vi "统计信息.vi"() -> ()   [LabVIEW 2016]
uses:
  <vilib>/Analysis/baseanly.llb/Mean (DBL).vi
  <vilib>/Analysis/NI_AALBase.lvlib
panel:
  in  "退出":bool
  out "表格":string[][](table)
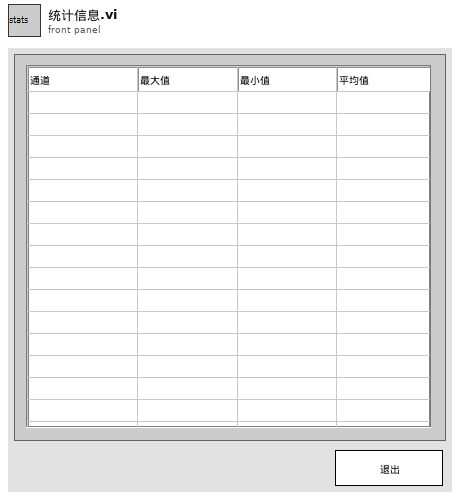
[diagram p1: front panel]
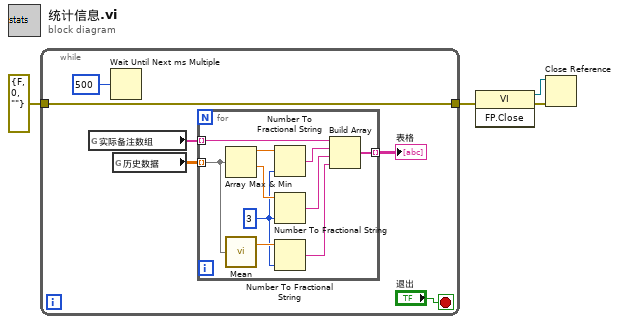
[diagram p0: block diagram]
diagram:
  n1 = while {
    tunnel: [w9] -> w2
    tunnel: errorcluster {"status"=FALSE, "code"=0, "source"=""} ("错误输出") -> [w9]
    stop <- "退出" stop-if-true
    n2 = global read "统计全局变量.vi" "实际备注数组"() -> (w8:string[])
    n3 = Wait Until Next ms Multiple(millisecond multiple=u32 500 ("毫秒倍数")) -> ()  [unwired: 1 out]
    n4 = global read "统计全局变量.vi" "历史数据"() -> (w5:sgl[][])
    n5 = for {
      tunnel: w8 -> [w17] mode=indexing
      tunnel: [w13] -> w7 mode=indexing
      tunnel: w5 -> [w11] mode=indexing
      w12 = i16 3 ("精度(6)")
      n6 = Array Max & Min(array=w11) -> (max value=w20:sgl, min value=w19:sgl)  [unwired: 2 out]
      n7 = call-poly <vilib>:"Mean.vi"("X"=w11) -> ("mean"=w18:dbl)  [unwired: 1 out]
      n8 = Number To Fractional String(number=w20, precision (6)=w12) -> (F-format string=w16:string)  [unwired: 2 in]
      n9 = Number To Fractional String(number=w19, precision (6)=w12) -> (F-format string=w15:string)  [unwired: 2 in]
      n10 = Number To Fractional String(number=w18, precision (6)=w12) -> (F-format string=w14:string)  [unwired: 2 in]
      n11 = Build Array(w17, w16, w15, w14) -> (w13:string[])
    }
    "表格" <- w7
  }
  n12 = invoke class="VI" method="FP.Close"(error in=w2) -> (reference out=w4:refnum<vi>, error out=w3:errorcluster)  [unwired: 2 in, 1 out]
  n13 = Close Reference(reference=w4, error in (no error)=w3) -> ()  [unwired: 1 out]
